vi "Test Process Request Returns on Error.vi"(8 "error in (no error)":errorcluster, 11 "Process Test In":refnum<class "Process Dev Test.lvclass">) -> (0 "error out":errorcluster, 3 "Process Test Out":refnum<class "Process Dev Test.lvclass">)   [LabVIEW 2020, in "Process Dev Test.lvclass"]
uses:
  Process Dev Test.lvclass
  C:/Program Files (x86)/National Instruments/LabVIEW 2020/vi.lib/Astemes/LUnit/Test Case.lvclass
  source/Framework Test Suite/Mock Process/Mock Process.lvclass
  C:/Git/astemes-triarc-framework/source/Framework/Process/Process.lvclass
  <vilib>/Astemes/LUnit/Test Case.lvclass/Test Case.ctl
  <vilib>/Astemes/LUnit/LUnit Assertion Result.lvclass/LUnit Assertion Result.ctl
  <vilib>/Astemes/LUnit/LUnit Test Case Result.lvclass/LUnit Test Case Result.ctl
  <vilib>/Astemes/LUnit/LUnit Method Result.lvclass/LUnit Method Result.ctl
  source/Framework/Process/Process.lvclass/Process.ctl
  <vilib>/Astemes/LUnit/Palette/Fail.vi
  <vilib>/Astemes/LUnit/Palette/Pass.vi
  <vilib>/Astemes/LUnit/Set Assertion Type.vi
  <vilib>/Astemes/LUnit/Palette/Pass If Equal.vi/cbf50e99-f124-4847-863a-8e9794d3dede.vi
  source/Framework/Process/Private/SubVIs/Wait for finish.vi
  source/Framework/Process/Protected/Messaging/Enqueue Message.vi
  source/Framework/Process/Private/SubVIs/Set Lifecycle State.vi
  source/Framework/Process/Public/Lifecycle/Get Lifecycle State.vi
  <vilib>/Astemes/LUnit/Add test result.vi
  <vilib>/Astemes/LUnit/LUnit Write Passed.vi
  <vilib>/Astemes/LUnit/LUnit Write Message.vi
  <vilib>/Astemes/LUnit/LUnit Write Description.vi
  <vilib>/Astemes/LUnit/LUnit Write Assertion Type.vi
  <vilib>/Astemes/LUnit/Compare Variants.vi
  <vilib>/Astemes/LUnit/Describe Comparison.vi
  source/Framework/Process/Private/SubVIs/Handle Debug Data.vi
  <vilib>/Utility/error.llb/Clear Errors.vi
  <vilib>/Astemes/LUnit/LUnit Record Assertion Result.vi
  <vilib>/Astemes/LUnit/Variant to string.vi
  source/Framework/Logging/Log Debug.vi
  <vilib>/AdvancedString/1D String Array to Delimited String.vi
  <vilib>/Utility/High Resolution Relative Seconds.vi
  <vilib>/Astemes/LUnit/LUnit Aggregate Assertion Results.vi
  <vilib>/Astemes/LUnit/Assertion Result/LUnit Read Status.vi
  <vilib>/Astemes/LUnit/LUnit Read Message.vi
  <vilib>/Astemes/LUnit/LUnit Read Description.vi
  <vilib>/Astemes/LUnit/Method Result/LUnit Merge Status.vi
  <vilib>/Astemes/LUnit/LUnit Concatenate result strings.vi
  <vilib>/Utility/error.llb/Error Cluster From Error Code.vi
  <vilib>/Utility/Data Type/Get Type Information.vi
  <vilib>/Utility/LVClass/Get LV Class Name.vi
  source/Framework/Process/Public/Read Name.vi
  <vilib>/ErrorRing/Error Ring.xnode
  <vilib>/Astemes/LUnit/LUnit Assertion Result.lvclass
  source/Framework/Process/Process.lvclass
  <vilib>/Astemes/LUnit/Test Case.lvclass
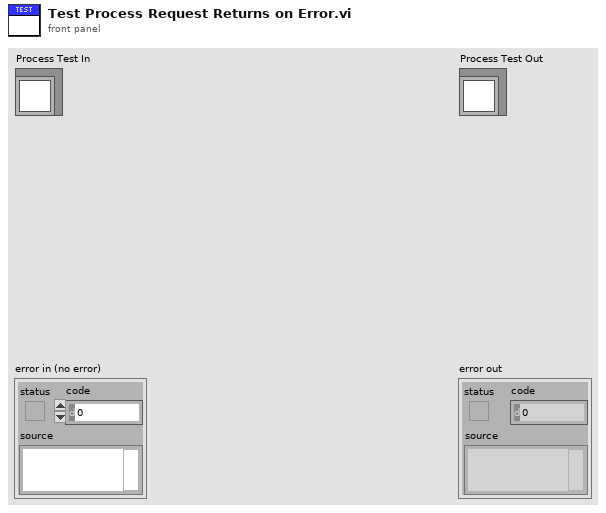
[diagram p1: front panel]
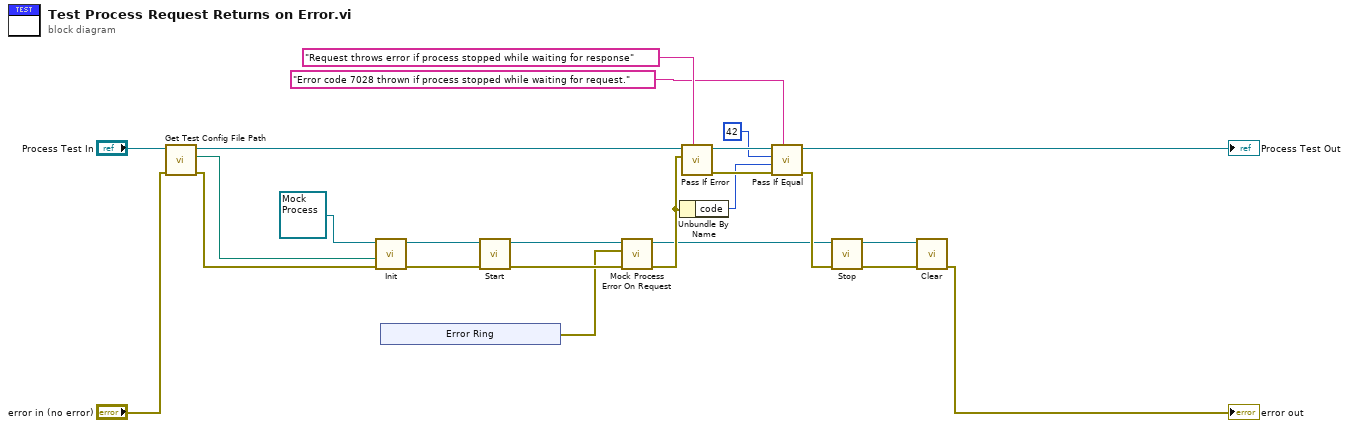
[diagram p0: block diagram]
diagram:
  n1 = call "Get Test Config File Path.vi"("error in (no error)"="error in (no error)", "Process Test In"="Process Test In") -> ("error out"=w17:errorcluster, "Test config path"=w18:path, "Process Test Out"=w20:refnum<class "Process Dev Test.lvclass">)  [unwired: 7 in]
  n2 = call-dynamic "Init.vi"("error in (no error)"=w17, "Config File Path"=w18, "Mock Process In"=refnum<class "Mock Process.lvclass"> refnum ("Mock Process.lvclass")) -> ("error out"=w21:errorcluster, "Mock Process Out"=w22:refnum<class "Mock Process.lvclass">)  [unwired: 7 in]
  n3 = xnode "Error Ring"() -> ("error out"=w5:errorcluster)
  n4 = call "Start.vi"("error in (no error)"=w21, "Process In"=w22) -> ("error out"=w14:errorcluster, "Process Out"=w2:refnum<class "Mock Process.lvclass">)  [unwired: 7 in, 1 out]
  n5 = call "Mock Process Error On Request.vi"("error in (no error)"=w14, "Mock Error"=w5, "Mock Process in"=w2) -> ("error out"=w9:errorcluster, "Mock Process out"=w1:refnum<class "Mock Process.lvclass">)  [unwired: 7 in]
  n6 = Unbundle By Name(w9) -> ("code"=w8:i32)
  n7 = call <vilib>:"Pass If Error.vi"("Description"="Request throws error if process stopped while waiting for response", "Assert error"=w9, "LUnit Test Case In"=w20) -> ("error out"=w10:errorcluster, "LUnit Test Case Out"=w13:refnum<class "Process Dev Test.lvclass">)  [unwired: 7 in]
  n8 = call <vilib>:"Pass If Equal.vi"("Description"="Error code 7028 thrown if process stopped while waiting for request.", "error in (no error)"=w10, "Actual"=w8, "Expected"=42 ("code"), "LUnit Test Case In"=w13) -> ("error out"=w4:errorcluster, "LUnit Test Case Out"=→"Process Test Out":refnum<class "Process Dev Test.lvclass">)  [unwired: 5 in]
  n9 = call "Stop.vi"("error in (no error)"=w4, "Process In"=w1) -> ("error out"=w3:errorcluster, "Process Out"=w24:refnum<class "Mock Process.lvclass">)  [unwired: 7 in, 1 out]
  n10 = call-dynamic "Clear.vi"("error in (no error)"=w3, "Mock Process In"=w24) -> ("error out"=→"error out":errorcluster)  [unwired: 9 in]
